vi "SUB-여러줄 문자열을 배열로 변환.vi"(1 "문자열":string) -> (0 "배열":string[](array[string]))   [LabVIEW 2011]
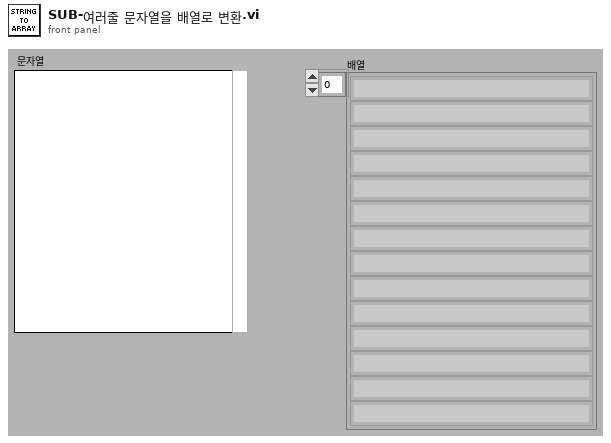
[diagram p1: front panel]
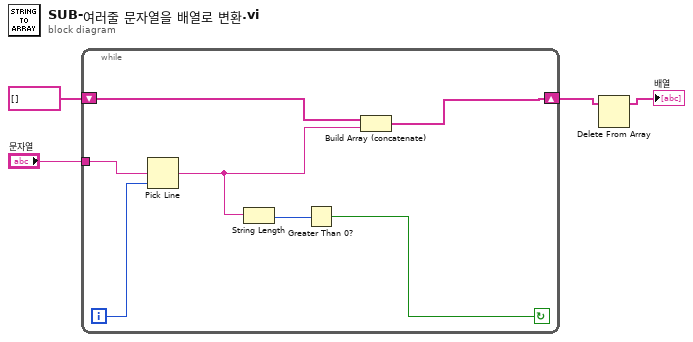
[diagram p0: block diagram]
diagram:
  n1 = while {
    tunnel: "문자열" -> [w11]
    shift-right: [w9] -> w2
    shift-left: string[] [] -> [w10]
    i -> [w8]
    stop <- w5 continue-if-true
    n2 = Pick Line(multi-line string=w11, line index=w8) -> (output string=w7:string)  [unwired: 1 in]
    n3 = String Length(string=w7) -> (length=w6:i32)
    n4 = Greater Than 0?(x=w6) -> (x > 0?=w5:bool)
    n5 = Build Array (concatenate)(w10, w7) -> (w9:string[])
  }
  n6 = Delete From Array(array=w2) -> (array with subset deleted=→"배열":string[])  [unwired: 2 in, 1 out]
